vi "week9_paddlewheel-V-to-steps_subVI.vi"(0 "DAQmx Device Name":tag="Dev1", 1 "V-threshold [V]":dbl=-1.2) -> ()   [LabVIEW 2019]
uses:
  <vilib>/measure/matone.llb/Extract Single Tone Information N Chan.vi
  <vilib>/measure/NI_MAPro.lvlib
panel:
  in  "Traditional DAQ Channel":tag
  in  "Averaging time [s]":dbl=3.0
  out "FFT Hz":dbl format="%_3g"
  out "Paddlewheel voltage":dynamicdata(graph)
  out "Hz":dbl format="%_3g"
  in  "# Steps":dbl format="%_4g"
  # "K-factor = coefficient to convert paddlewheel frequency to flow rate\nAveraging time = time over which to obtain paddlewheel V readings\nV-threshold = Voltage threshold used to count a step change / paddlewheel rotation. Set this value to a voltage intermediated between the paddlewheel max. and min. voltages"
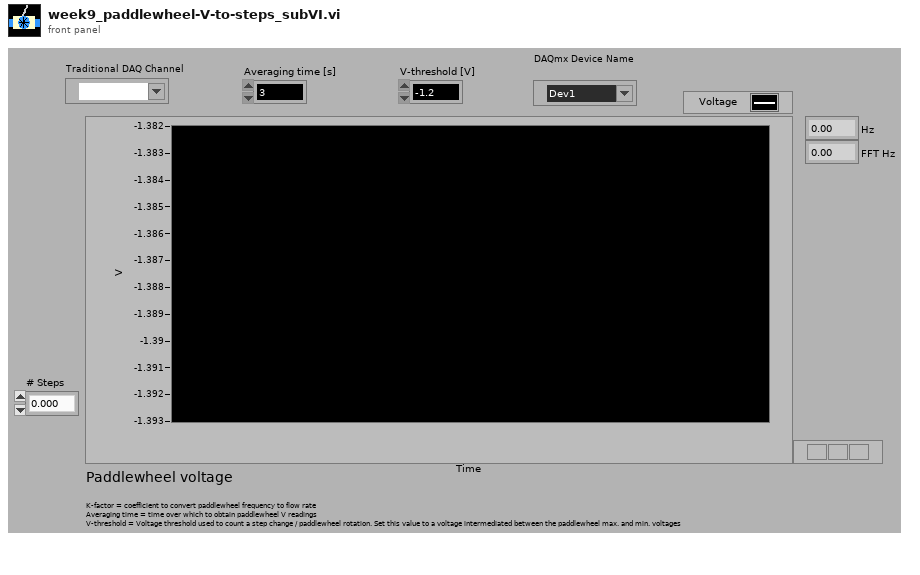
[diagram p1: front panel]
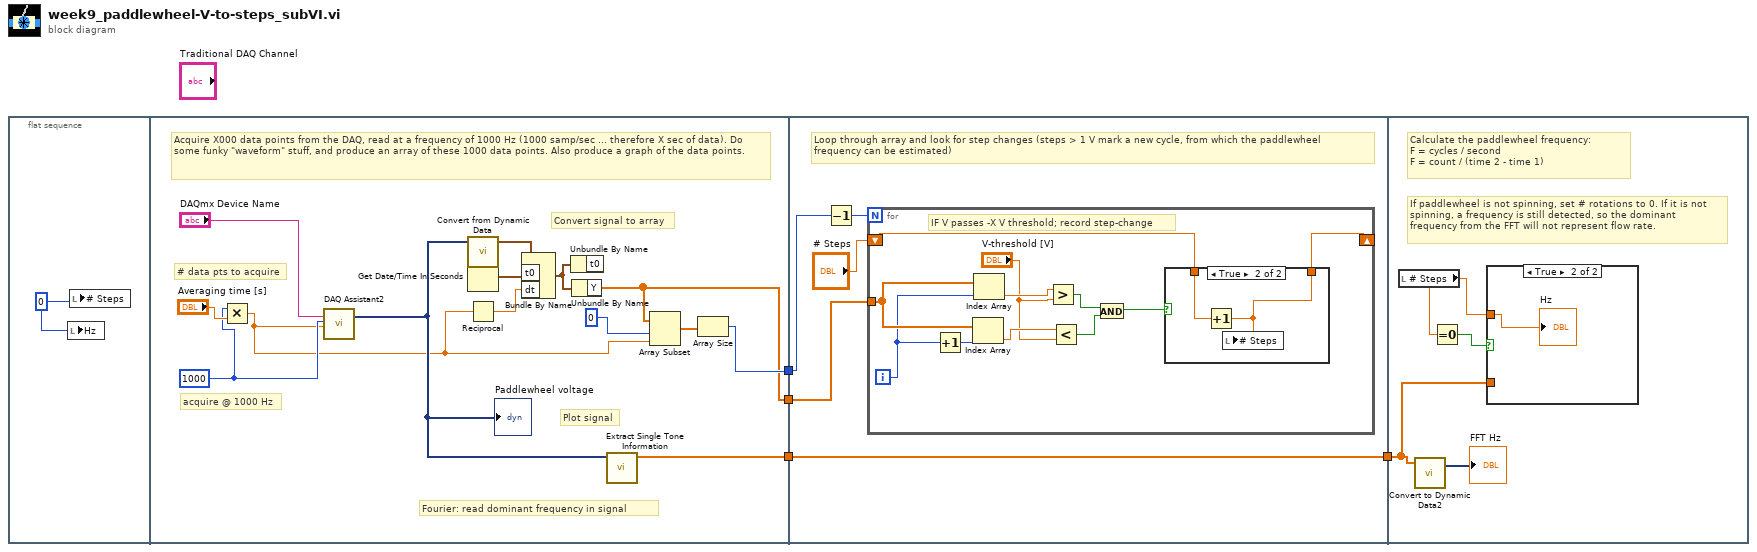
[diagram p0: block diagram]
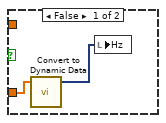
[diagram p3: hidden frame]
diagram:
  n1 = flat-sequence {
    tunnel: [w13] -> w3
    tunnel: [w9] -> w2
    tunnel: [w11] -> w1
    tunnel: w3 -> [w24]
    tunnel: w2 -> [w22]
    tunnel: w1 -> [w20]
    tunnel: [w20] -> w4
    tunnel: w4 -> [w39]
    frame #0 {
      w5 = 0
      n2 = local write "Hz"(w5) -> ()
      n3 = local write "# Steps"(w5) -> ()
    }
    frame #1 {
      w7 = 1000
      # "Plot signal"
      # "Convert signal to array"
      # "acquire @ 1000 Hz"
      # "# data pts to acquire"
      # "Fourier: read dominant frequency in signal"
      # "Acquire X000 data points from the DAQ, read at a frequency of 1000 Hz (1000 samp/sec ... therefore X sec of data). Do some funky \"waveform\" stuff, and produce an array of these 1000 data points. Also produce a graph of the data points."
      n4 = Multiply(x=w7, y="Averaging time [s]") -> (x*y=w6:dbl)
      n5 = call "DAQ Assistant2"("rate"=w7, "number of samples"=w6, "device name"="DAQmx Device Name") -> ("data"=w12:dynamicdata)  [unwired: 14 in, 2 out]
      "Paddlewheel voltage" <- w12
      n6 = call "Convert from Dynamic Data"("Dynamic Data Type"=w12) -> ("Waveform"=w14:waveform(dbl))  [unwired: 3 in]
      n7 = Get Date/Time In Seconds() -> (seconds since 1Jan1904=w15:timestamp)
      n8 = Reciprocal(x=w6) -> (1/x=w16:dbl)
      n9 = Bundle By Name(cluster=w14, "t0"=w15, "dt"=w16) -> (w17:waveform(dbl))
      n10 = Unbundle By Name(w17) -> ()  [unwired: 1 out]
      n11 = Unbundle By Name(w17) -> ("Y"=w9:dbl[])
      n12 = call-poly <vilib>:"Extract Single Tone Information.vi"("time signals in"=w12) -> ("detected frequencies"=w11:dbl[])  [unwired: 5 in, 5 out]
      n13 = Array Subset(array=w9, index=0, length=w6) -> (w19:dbl[])
      n14 = Array Size(array=w19) -> (size(s)=w13:i32)
    }
    frame #2 {
      # "Loop through array and look for step changes (steps > 1 V mark a new cycle, from which the paddlewheel \nfrequency can be estimated)"
      n15 = Decrement(x=w24) -> (x-1=w23:i32)
      n16 = for {
        N: w23 -> [_]
        shift-right: [w35] -> _
        shift-left: "# Steps" -> [w31]
        tunnel: w22 -> [w34]
        i -> [w33]
        # "IF V passes -X V threshold; record step-change"
        n17 = Increment(x=w33) -> (x+1=w32:i32)
        n18 = Index Array(array=w34, index=w32) -> (element=w27:dbl)
        n19 = Index Array(array=w34, index=w33) -> (element=w26:dbl)
        n20 = Greater?(x=w26, y="V-threshold [V]") -> (0:w30:bool)
        n21 = Less?(x=w27, y="V-threshold [V]") -> (x < y?=w28:bool)
        n22 = And(x=w30, y=w28) -> (x .and. y?=w29:bool)
        n23 = case shown="True" w29 {
          tunnel: [w36 w37] -> w35
          tunnel: w31 -> [w36 w38]
          frame False {
          }
          frame True {
            n24 = Increment(x=w38) -> (x+1=w37:dbl)
            n25 = local write "# Steps"(w37) -> ()
          }
        }
      }
    }
    frame #3 {
      # "If paddlewheel is not spinning, set # rotations to 0. If it is not spinning, a frequency is still detected, so the dominant\nfrequency from the FFT will not represent flow rate."
      # "Calculate the paddlewheel frequency:\nF = cycles / second\nF = count / (time 2 - time 1)"
      n26 = local read "# Steps"() -> (w41:dbl)
      n27 = call "Convert to Dynamic Data2"("Array"=w39) -> ("Dynamic Data Type"=→"FFT Hz":dynamicdata)  [unwired: 3 in]
      n28 = Equal To 0?(x=w41) -> (x = 0?=w42:bool)
      n29 = case shown="True" w42 {
        tunnel: w41 -> [_ w45]
        tunnel: w39 -> [w44 _]
        frame False {
          n30 = call "Convert to Dynamic Data"("Array"=w44) -> ("Dynamic Data Type"=w43:dynamicdata)  [unwired: 3 in]
          n31 = local write "Hz"(w43) -> ()
        }
        frame True {
          "Hz" <- w45
        }
      }
    }
  }
